vi "Initialize MeasIndices in Visulaization Properties Control.vi"(8 "error in (no error)":errorcluster, 10 "MeasChannels":string[](array[string]), 11 "VisualizationProperties":T1={"PauseAtStartup"=TRUE, "LogData"=FALSE, "LaunchInSubPanel"=TRUE, "FPMonitor"=0, "FPWindowBounds"={"Left"=0, "Top"=0, "Right"=0, "Bottom"=0}, "MonitorBounds"={"Left"=0, "Top"=0, "Right"=0, "Bottom"=0}, "MeasIndices"=[]}) -> (0 "error out":errorcluster, 3 "VisualizationProperties out":T1={"PauseAtStartup"=TRUE, "LogData"=FALSE, "LaunchInSubPanel"=TRUE, "FPMonitor"=0, "FPWindowBounds"={"Left"=0, "Top"=0, "Right"=0, "Bottom"=0}, "MonitorBounds"={"Left"=0, "Top"=0, "Right"=0, "Bottom"=0}, "MeasIndices"=[]})   [LabVIEW 2018, in "Visualization.lvlib" / "VisualizeSensor.lvclass"]
uses:
  Sensor/VisualizeSensor.lvclass
  VisualizationOptions.ctl
  <vilib>/Utility/miscctls.llb/LVRectTypeDef.ctl
  VisualizeBase.lvclass
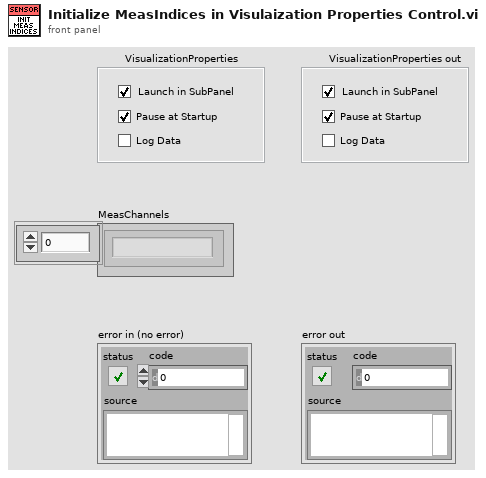
[diagram p1: front panel]
types:
  T1 = typedef "Visualization.lvlib/VisualizeBase.lvclass/VisualizationOptions.ctl" = cluster{"PauseAtStartup":bool, "LogData":bool, "LaunchInSubPanel":bool, "FPMonitor":u16, "FPWindowBounds":T2, "MonitorBounds":cluster{"Left":i16, "Top":i16, "Right":i16, "Bottom":i16}, "MeasIndices":i32[]}
  T2 = typedef "LVRectTypeDef.ctl" = cluster{"Left":i16, "Top":i16, "Right":i16, "Bottom":i16}
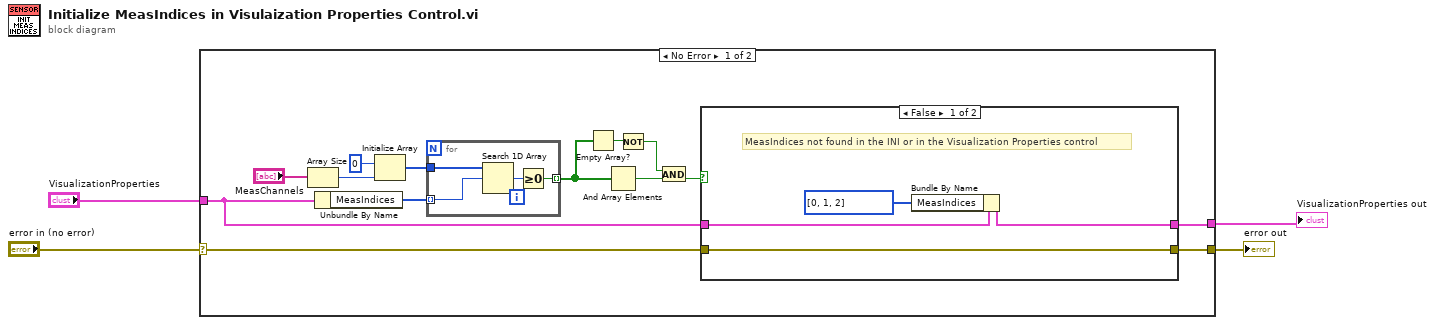
[diagram p0: block diagram]
diagram:
  n1 = case shown="No Error" "error in (no error)" {
    selector: "error in (no error)" -> [w6 w30]
    tunnel: "VisualizationProperties" -> [w16 w29]
    tunnel: [w7 w30] -> w3
    tunnel: [w5 w29] -> w1
    frame No Error {
      n2 = Array Size(array="MeasChannels") -> (size(s)=w14:i32)
      n3 = Unbundle By Name(w16) -> ("MeasIndices"=w17:i32[])
      n4 = Initialize Array(0, w14) -> (w12:i32[])
      n5 = for {
        tunnel: w17 -> [w21] mode=indexing
        tunnel: w12 -> [w22]
        tunnel: [w19] -> w11 mode=indexing
        n6 = Search 1D Array(1D array=w22, element=w21) -> (index of element=w20:i32)  [unwired: 1 in]
        n7 = Greater Or Equal To 0?(x=w20) -> (x >= 0?=w19:bool)
      }
      n8 = Empty Array?(array=w11) -> (empty?=w10:bool)
      n9 = And Array Elements(Boolean array=w11) -> (logical AND=w18:bool)
      n10 = Not(x=w10) -> (.not. x?=w8:bool)
      n11 = And(x=w8, y=w18) -> (x .and. y?=w9:bool)
      n12 = case shown="False" w9 {
        tunnel: w16 -> [w26 w27]
        tunnel: w6 -> [w23 w28]
        tunnel: [w23 w28] -> w7
        tunnel: [w24 w27] -> w5
        frame False {
          # "MeasIndices not found in the INI or in the Visualization Properties control"
          n13 = Bundle By Name(cluster=w26, "MeasIndices"=i32[] [0, 1, 2]) -> (w24:T1)
        }
        frame True {
        }
      }
    }
    frame Error {
    }
  }
  "error out" <- w3
  "VisualizationProperties out" <- w1
